vi "Filter Classes Descending from Test Case.vi"(8 "error in (no error)":errorcluster, 11 "Project Items":refnum<vi>[](array[refnum])) -> (0 "error out":errorcluster, 3 "Project Items out":refnum<vi>[](array[refnum]))   [LabVIEW 2020, in "Coverage Analyzer.lvlib" / "Coverage Analyzer.lvclass"]
uses:
  Coverage Analyzer.lvclass
  LUnit Test Case.lvclass
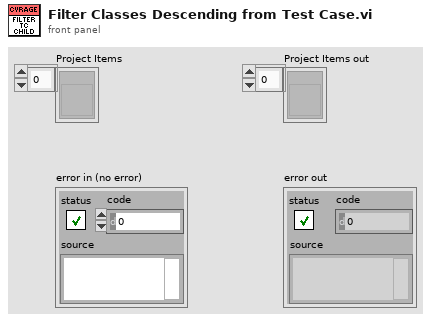
[diagram p1: front panel]
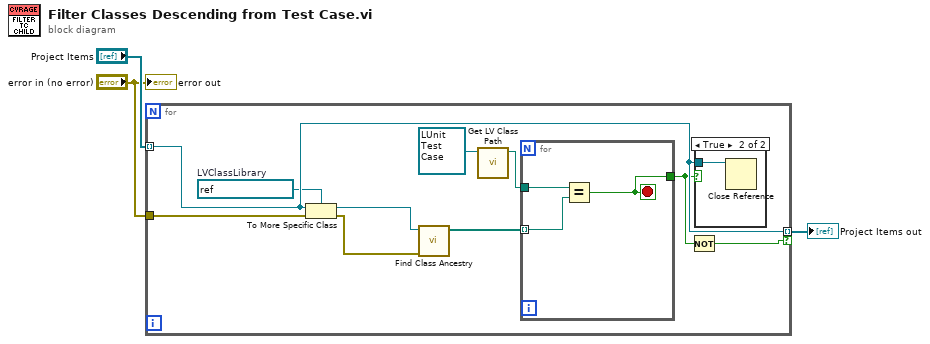
[diagram p0: block diagram]
diagram:
  n1 = for {
    tunnel: "Project Items" -> [w12] mode=indexing
    tunnel: "error in (no error)" -> [w13]
    tunnel: [w12] -> w1 mode=indexing if=w10
    w9 = refnum<vi> refnum  # LVClassLibrary
    n2 = To More Specific Class(target class=w9, reference=w12, error in=w13) -> (specific class reference=w6:refnum<vi>, error out=w4:errorcluster)
    n3 = call "Find Class Ancestry.vi"("error in (no error)"=w4, "reference in"=w6) -> ("Class Ancestry"=w5:path[])  [unwired: 8 in, 1 out]
    n4 = call <vilib>:"Get LV Class Path.vi"("object"=refnum<class "LUnit Test Case.lvclass"> refnum ("LUnit Test Case V2.lvclass")) -> ("class path"=w8:path)  [unwired: 9 in, 1 out]
    n5 = for {
      tunnel: [w15] -> w11
      tunnel: w5 -> [w16] mode=indexing
      tunnel: w8 -> [w14]
      stop <- w15 stop-if-true
      n6 = Equal?(x=w14, y=w16) -> (x = y?=w15:bool)
    }
    n7 = Not(x=w11) -> (.not. x?=w10:bool)
    n8 = case shown="True" w11 {
      tunnel: w12 -> [_ w17]
      frame False {
      }
      frame True {
        n9 = Close Reference(reference=w17) -> ()  [unwired: 1 in, 1 out]
      }
    }
  }
  "Project Items out" <- w1
  "error out" <- "error in (no error)"
